vi "DIAdem Restart Variables.vi"() -> (1 "Restart enabled?":bool, 2 "TIME (24hr)":string, 3 "Needs Restart?":bool)   [LabVIEW 2011]
uses:
  ITK EXT/utils/strutil.llb/Case Matching.ctl
  server lib/Spartan CONFIG Global.vi
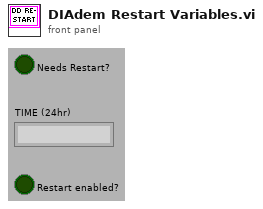
[diagram p1: front panel]
types:
  T1 = typedef "Case Matching.ctl" = enum16{"a != A", "a == A", "system"}
  T2 = typedef "Keyed Array.ctl" = cluster{"keys":string[], "values":string[]}
  T3 = typedef "LVDateTimeRec.ctl" = cluster{"fractional second":dbl, "second":i32, "minute":i32, "hour":i32, "day of month":i32, "month":i32, "year":i32, "day of week":i32, "day of year":i32, "DST":i32}
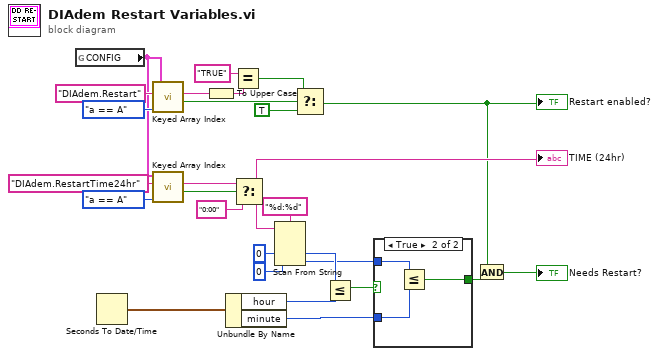
[diagram p0: block diagram]
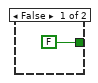
[diagram p2: hidden frame]
diagram:
  n1 = global read "Spartan CONFIG Global.vi" "CONFIG"() -> (w23:T2)
  n2 = Seconds To Date/Time() -> (date time rec=w13:T3)  [unwired: 2 out]
  n3 = call "Keyed Array Index.vi"("case matching (sensitive)"=Case_Matching."a == A", "key"="DIAdem.Restart", "array in"=w23) -> ("valid key"=w22:bool, "value"=w21:string)  [unwired: 1 in, 2 out]
  n4 = call "Keyed Array Index.vi"("case matching (sensitive)"=Case_Matching."a == A", "key"="DIAdem.RestartTime24hr", "array in"=w23) -> ("valid key"=w16:bool, "value"=w15:string)  [unwired: 1 in, 2 out]
  n5 = To Upper Case(1:w21) -> (0:w19:string)
  n6 = Unbundle By Name(w13) -> ("hour"=w7:i32, "minute"=w4:i32)
  n7 = Equal?(x="TRUE", y=w19) -> (x = y?=w20:bool)
  n8 = Select(t=w15, s=w16, f="0:00" ("x")) -> (s? t:f=w12:string)
  "TIME (24hr)" <- w12
  n9 = Scan From String(format string="%d:%d", input string=w12, default 1=0 ("default value 1"), default 2=0 ("default value 2")) -> (output 1=w8:i32, output 2=w5:i32)  [unwired: 2 in, 3 out]
  n10 = Select(t=w20, s=w22, f=TRUE) -> (s? t:f=w2:bool)
  "Restart enabled?" <- w2
  n11 = Less Or Equal?(x=w8, y=w7) -> (x <= y?=w6:bool)
  n12 = case shown="True" w6 {
    tunnel: w5 -> [_ w31]
    tunnel: w4 -> [_ w30]
    tunnel: [FALSE w29] -> w3
    frame False {
    }
    frame True {
      n13 = Less Or Equal?(x=w31, y=w30) -> (x <= y?=w29:bool)
    }
  }
  n14 = And(x=w2, y=w3) -> (x .and. y?=→"Needs Restart?":bool)
